vi "Post-Build Action.vi"(5 "files generated by build":path[](array[path]), 6 "top level/always included VIs":path[](array[path]), 7 "destination path":path, 8 "error in":errorcluster, 9 "target name":string, 10 "build specification name":string, 11 "project path":path) -> (0 "error out":errorcluster)   [LabVIEW 2025, in "WorkflowDO.lvclass"]
uses:
  WorkflowDO.lvclass
  WorkflowDO.lvclass/WorkflowDO.ctl
  C:/Program Files/National Instruments/LabVIEW 2025/vi.lib/Plug-In SDKs/Measurements/Measurement Plugin Service/Measurement Plugin Service.lvclass
  C:/Users/Administrator/Documents/ggonzalez/hardware-validation/src/labview/workflow-can/WorkflowDO/WorkflowDO.lvclass
  <vilib>/Plug-In SDKs/Measurements/NI Measurement Plug-In SDK.lvlib
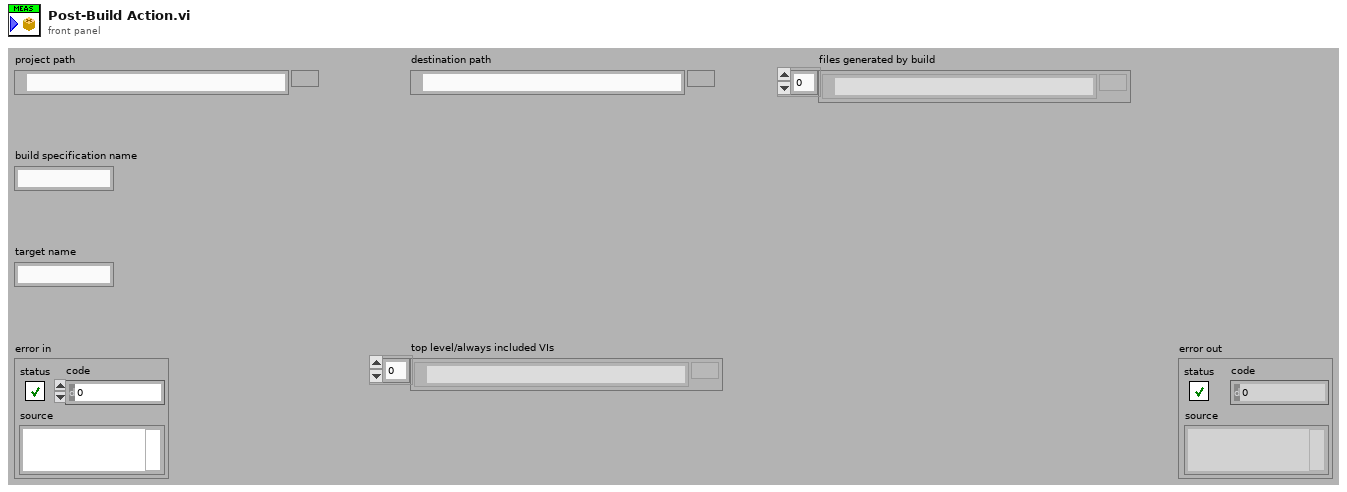
[diagram p1: front panel]
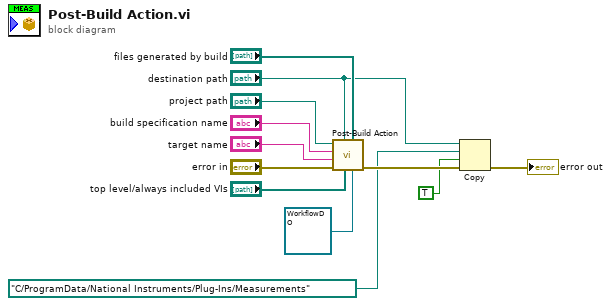
[diagram p0: block diagram]
diagram:
  n1 = call <vilib>:"Post-Build Action.vi"("measurement plugin service"=refnum<class "WorkflowDO.lvclass"> refnum ("MeasurementLink Measurement Template.lvlib:MeasurementPlugin.lvclass"), "files generated by build"="files generated by build", "top level/always included VIs"="top level/always included VIs", "destination path"="destination path", "error in"="error in", "target name"="target name", "build specification name"="build specification name", "project path"="project path") -> ("error out"=w11:errorcluster)  [unwired: 3 in]
  n2 = Copy(8:w11, 9:TRUE ("overwrite (F)"), 10:path "C:/ProgramData/National Instruments/Plug-Ins/Measurements" ("target path (use dialog)"), 11:"destination path") -> (0:→"error out":errorcluster)  [unwired: 1 in, 2 out]
